vi "AlliGator Send Local Decay Plots.vi"(8 "error in (no error)":errorcluster, 10 "ROI Descriptor":T1 {"Contours"."Type" items=["No Selection", "Point", "Line", "Rectangle", "Oval", "Polygon", "Freehand Region", "Annulus", "Unused2", "Unused3", "Broken Line", "Freehand Line", "Rotated Rectangle"]}, 11 "AlliGator IV DVR in":refnum<data-value>) -> (0 "error out":errorcluster, 3 "AlliGator IV DVR out":refnum<data-value>)   [LabVIEW 2021, in "AlliGator Local Decay Window.lvlib"]
doc: "Gets the data (decay, fit, IRF, residuals and fit parameters) at the selected ROI and sends it to the Local Decay Window for update."
uses:
  AlliGator Local Decay Window.lvlib
  Internal Variables/AlliGator Internal Variables v2.ctl
  <vilib>/vision/Image Controls.llb/IMAQ Image.ctl
  Internal Variables/AlliGator Gate Image Set.ctl
  Files/AlliGator FLI Dataset Type.ctl
  Files/AlliGator Data Series Type.ctl
  Dual-Channel Datasets/AlliGator Dataset Channel.ctl
  Settings/AlliGator Gate Arithmetic.ctl
  Source Image/AlliGator Displayed Image.ctl
  Image/Named ROI Description.ctl
  Phasor Graph/AlliGator Decay Metadata v3.ctl
  Decay Analysis/Decay Preprocessing/AlliGator Decay Background Subtraction Info.ctl
  Decay Analysis/Decay Preprocessing/AlliGator Baseline Subtraction Method.ctl
  Graphs/XY Graph/XY Graph Plot Shift Parameters.ctl
  Graphs/XY Graph/XY Graph Plot Shift Method.ctl
  Decay Analysis/Decay Preprocessing/AlliGator Decay Extrapolation Parameters.ctl
  Phasor/Calibration Phasor (m, phi).ctl
  Phasor/Phasor Reference Series.ctl
  Phasor/Phasor Calibration Map v2.ctl
  Phasor/Phasor (g, s).ctl
  Phasor Graph/AlliGator Raw Phasor Plot Data v5.ctl
  Phasor/Phasor Standard Deviation Options.ctl
  Phasor Plot/AlliGator Phasor Multi-Harmonic Data.ctl
  Phasor/Phasor Harmonic Data.ctl
  Decay Fit Parameter Map/AlliGator Decay Fit Options & Parameters v4.ctl
  Fits/IRF(X)PSED/Decay Fit Options v4.ctl
  Fits/Decay Convolution/Decay Model.ctl
  Fits/Residual Type.ctl
  Fits/IRF(X)PSED/Fit Weights Type v2.ctl
  Fits/Non-linear Fitting Method v2.ctl
  Fits/Fit Calculation Method.ctl
  Fits/Non-linear Fitting Algorithm.ctl
  Decay Analysis/Decay Fit/AlliGator Decay Fit Parameter Constraints 2.ctl
  Fits/IRF(X)PSED/Decay Fit Parameters In List.ctl
  Fits/IRF(X)PSED/MLE Baseline Offset Type.ctl
  Decay Analysis/Decay Preprocessing/AlliGator Decay Preprocessing Parameters.ctl
  Fits/IRF(X)PSED/Decay Fit Parameters & Derived Quantities List v2.ctl
  Fits/IRF(X)PSED/Decay Fit Result Constraint.ctl
  Decay Fit Parameter Map/AlliGator Parameter Maps Data.ctl
  Globals, Variables, Constants/AlliGator Variables List.ctl
  AlliGator Local Decay Graph Window Event Refnum.ctl
  AlliGator Local Decay Fit Results.ctl
  Image Profile Window/AlliGator Image Profile Plot Data.ctl
  Graphs/XY Graph/XY Graph Plot Data.ctl
  Utilities/Read-Write.ctl
  Variant/Variant to Data/Variant to U16.vi
  Variant/Variant to Data/Variant to Boolean.vi
  Globals, Variables, Constants/AlliGator Globals, Variables & Constants.lvlib
  Graphs/XY Graph/XY Graph Add-Ons.lvlib
  Image Profile Window/AlliGator Image Profile Window.lvlib
  Decay Analysis/Decay Processing/AlliGator Decay Processing.lvlib
  Time/Time.lvlib
  Decay Fit Parameter Map/AlliGator Decay Fit Parameter Map.lvlib
  Decay Analysis/Decay Preprocessing/AlliGator Decay Preprocessing.lvlib
  GUI/AlliGator GUI.lvlib
  Utilities/Utilities.lvlib
  Variant/Variant to Data/Variant to Data.lvlib
  Image/Image.lvlib
  Fits/Fits.lvlib
  Phasor/Phasor.lvlib
  Internal Variables/AlliGator Internal Variables.lvlib
  Files/AlliGator Files.lvlib
  Phasor Graph/AlliGator Phasor Graph.lvlib
  Phasor Plot/AlliGator Phasor Plot.lvlib
  Source Image/AlliGator Source Image.lvlib
  Decay Analysis/Decay Fit/AlliGator Decay Fit.lvlib
  Settings/AlliGator Settings.lvlib
  Dual-Channel Datasets/AlliGator Dual-Channel Datasets.lvlib
panel:
  out "CPU (s)":dbl
  # "see the AlliGator License on the block diagram (Ctrl+E or Window:Show Block Diagram)"
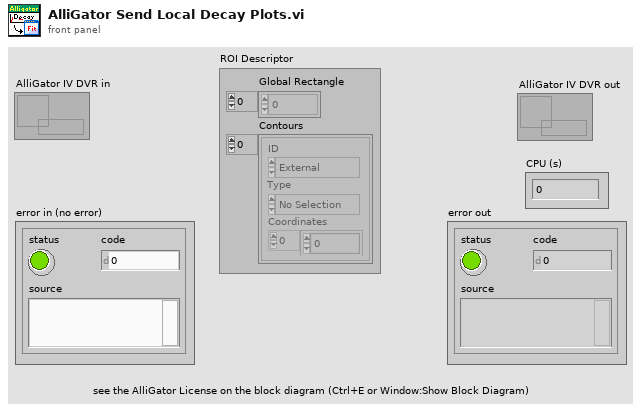
[diagram p1: front panel]
types:
  T1 = typedef "ROI Descriptor" = cluster{"Global Rectangle":i32[], "Contours":cluster{"ID":enum32{"External", "Internal"}, "Type":u32, "Coordinates":i32[]}[]}
  T2 = typedef "AlliGator Local Decay Window.lvlib/AlliGator Local Decay Graph Window Event Refnum.ctl" = refnum<user-event>
  T3 = typedef "AlliGator Globals, Variables & Constants.lvlib/AlliGator Variables List.ctl" = enum16{"---- GUI ----", "GUI:Initialization Status", "GUI:State Indicators Refnum", "GUI:Original AlliGator Menu Items", "GUI:Current Action Loop State", "GUI:Script in progress", "GUI:Playback", "GUI:Loop Playback", "GUI:Search ROI Used", "GUI:Search ROI", "Decay Graph Max Legend Size", "Intensity Graph Max Legend Size", "Decay Statistics Graph Max Legend Size", "Phasor Graph Max Legend Size", "Phasor Ratio Graph Max Legend Size", "Lifetime Graph Max Legend Size", "---- Files ----", "Files:Export Dataset Frames as Individual Files", "Files:Show Batch Export Help Balloons", "Files:Frames in Dataset", "Files:ptu File Frame Start Indices", "Files:Current Frame in Dataset", "Files:Current Frame Timestamp", "Files:Dataset Loaded", "Files:Dataset Metadata", "Files:Dataset Channel", "Files:Dataset Data Description", "Files:Background Dataset Metadata", "Files:Background Dataset Channel", "Files:Background Dataset Data Description", "Files:Background File Subtraction", "Files:Background File Path", "Files:Background File Pile-up Correction", "Files:Background File Pixel Well Capacity", "Files:Background File Scaling Factor", "Files:Current Dataset Load Settings", "Files:Dataset Path", "Files:ICCD-specific Information", "Files:Macrotime Gate Separation", "------ Python Plugins ------", "Python Plugins:Information", "Python Plugins:Python Session", "Python Plugins:Valid Python Session?", "---- Source Image ----", "Source Image:ROIs", "Source Image:Current ROI", "Source Image:ROI Event Refnum", "X_Source Image:Display Range", "X_Source Image:Palette Information", "X_Source Image:Type of Displayed Image", "X_Time Gate Slider", "Source Image:Palette List", "Source Image:Scale", "Source Image:ROI Overlay Color", "Source Image:Overlay to Erase", "Source Image:Is Displayed Image Accumulated", "Source Image:White Light Image Modified", "Source Image:Mask Image Modified", "---- Image Profile Window ----", "Image Profile:Window Event Refnum", "Image Profile:IntensityType", "Image Profile:Intensity Average Type", "Image Profile:Intensity-weighted SDV", "Image Profile:Box Profile Type", "Image Profile:Window Open", "Image Profile:Plotted Fit Parameter", "------ Phasor Graph -------", "Phasor Graph:Show Line", "---- Phasor Plot ---", "Phasor Plot:Parameters Changed", "Phasor Plot:FLI Dataset Modified since last Calculation", "Phasor Harmonics Data", "Selected Phasor Harmonics", "Phasor Harmonic Manager Event Refnum", "Phasor Plot:ROIs", "Phasor Plot:Current ROI", "Phasor Plot:ROI Event Refnum", "Phasor Plot:Image Reference Points", "Phasor Plot:Computed", "Phasor Plot:Palette Information", "Phasor Plot:Palette List", "Phasor Plot:Phasor Ratio Palette Information", "Phasor Plot:Phasor Ratio Palette List", "Phasor Plot:Image Scale", "Phasor Plot:Image Overlay to Erase", "Phasor Plot:Image Elements to Update", "Phasor Plot:Current Calculation Parameters", "Phasor Plot:Current Calibration Options", "Phasor Plot:Reset Cumulated Phasor Plot", "Phasor Plot:Reference 1", "Phasor Plot:Lifetime Reference 1", "Phasor Plot:Reference 1 Frequency", "Phasor Plot:Reference 2", "Phasor Plot:Lifetime Reference 2", "Phasor Plot:Reference 2 Frequency", "---- Decay Analysis ----", "Number of Selected Decays to Fit", "LS Fit Results", "LAR Fit Results", "BS Fit Results", "Last Decay Max - Min", "Best Fit Parameters", "Best Fit Parameter Names", "Actual Size X", "Actual Size Y", "Binning X", "Binning Y", "Actual # Gates", "Dataset Number", "Gates to...", "Gates Skipped", "Gates to keep", "Gate Step", "Gate Separation", "Reversed Gates", "Pile-up Correction", "Pixel Well Capacity", "Background Subtracted", "Background Subtraction Method", "Background Definition Range", "Background File (deprecated)", "Number of Dataset Accumulated", "Array of Accumulated Dataset Paths", "Do Averaged Datasets", "Destination File Path", "Process Plot Target", "Use 1/D as Phasor Frequency", "---- Decay Fit Parameter Map -----", "Decay Fit Parameter Map:Palette Information", "Decay Fit Parameter Map:Palette List", "Decay Fit Parameter Map:X Resolution", "Decay Fit Parameter Map:Y Resolution", "Decay Fit Parameter Map:Use Decay Fit Result Constraints", "Decay Fit Parameter Map:Decay Fit Result Constraints", "Decay Fit Parameter Map:Decay Fit Result Constraints Applied", "---- Parameter Map ----", "Parameter Map:Palette Information", "Parameter Map:Palette List", "------- Local Decay Window ---------", "Local Decay Graph Window:Event Refnum", "Local Decay Graph Window:Use normalized IRF for convolution", "----- Miscellaneous ----", "Misc:Skippable Dialog Windows Status"}
  T4 = typedef "IMAQ Image.ctl" = refnum<image>
  T5 = typedef "AlliGator Image Profile Window.lvlib/AlliGator Image Profile Plot Data.ctl" = cluster{"Plot Name":string, "Plot":T6}
  T6 = typedef "XY Graph Add-Ons.lvlib/XY Graph Plot Data.ctl" = cluster{"X Array":dbl[], "Y Array":dbl[]}
  T7 = typedef "AlliGator Internal Variables.lvlib/AlliGator Internal Variables v2.ctl" = cluster{"----------------------------- Images -----------------------------":u8, "Displayed Image":T4, "White Light Image":T4, "Mask Image":T4, "ROI Mask Image":T4, "Current Dataset Images 1":T8, "Background Dataset Images 1":T8, "Current Dataset Images 2":T8, "Background Dataset Images 2":T8, "Current Dataset Arithmetic Images":T8, "Accumulated Dataset Images 1":T8, "Accumulated Dataset Images 2":T8, "Accumulated Dataset Arithmetic Images":T8, "----------------------------- File Paths -----------------------------":u8, "Phasor Plot Image":T4, "Decay Fit Parameter Map Image":T4, "Parameter Map Image":T4, "Single Data Point Path":path, "White Light Image Path":path, "Mask Image Path":path, "Time-Series Folder":path, "[Time-Series Paths]":path[], "----------------------------- FLI Dataset -----------------------------":u8, "Current Dataset":i32, "Single Dataset Type":T9, "Current Folder":string, "AlliGator Data Series Type":T10, "# Datasets":i32, "Dual-Channel Dataset":bool, "Selected Channel Name":string, "Dataset Channel":T11, "Channel Arithmetic":T12, "Dual-Channel Background Dataset":bool, "Background Channel":T11, "Dual-Channel Accumulated Dataset":bool, "Start Time":dbl, "[Time-Series Timestamps]":dbl[], "[Intensity Corrections]":dbl[], "Time Series Script":bool, "Type of Displayed Image":T13, "Gate Image Slide":u16, "# Gates":i32, "ROIs":T14[], "----------------------------- Decays -----------------------------":u8, "ROI Decay":cluster{"t Array":dbl[], "I Array":dbl[]}, "Valid Decay":bool, "Decay  Metadata":T15, "Reference Decay Plot Name":string, "Reference Decay":cluster{"t Array":dbl[], "I Array":dbl[]}, "Decay Shift Plot":cluster{"Time Stamps":dbl[], "Decay Shifts":dbl[]}, "[Decays Max Values]":sgl[], "[Decays Min Values]":sgl[], "----------------------------- Calibration -----------------------------":u8, "Calibration Phasor":T21, "Calibration Phasor Series":T22, "Phasor Calibration Map":T23, "Calibration Map MD5 Digest":string, "----------------------------- Phasor Graph -----------------------------":u8, "Last Raw Phasor":T24, "Last Calibrated Phasor":T24, "Last Calibrated Phasor SDV":T24, "Phasor Graph:Phasor Plot":cluster{"g Array":dbl[], "s Array":dbl[]}, "Phasor Graph:Phasor SDV Plot":cluster{"g Array":dbl[], "s Array":dbl[]}, "[Phasor Graph:Raw Phasor Plots]":T25[], "Phasor Plot locked to Ref 1":i32, "[Phasor Plot(s) locked to Ref 1]":i32[], "[Phasor Plot(s) locked to Ref 2]":i32[], "[Pixel Phasors]":T24[], "----------------------------- Phasor Plot -----------------------------":u8, "[[Sum Image]]":dbl[][], "[[CSG Phasors]]":csg[][], "[[Valid Pixel?]]":bool[][], "[[Phasor Ratios]]":dbl[][], "[[Average Lifetimes]]":dbl[][], "Amplitude Weighted Average Lifetime":bool, "I/m/phi Dataset":cluster{"I/m/phi Dataset?":bool, "Base Frequency":dbl[unit], "Harmonic Orders":u8[]}, "Multi Phasor Plot Data":T27, "----------------------------- Decay Fit Parameter Map -----------------------------":u8, "Decay Fit Options & Parameters":T29, "Fit Options: Decay Preprocessing Parameters":T40, "Fit Options: Reference Decay":cluster{"t Array":dbl[], "I Array":dbl[]}, "Is Full Image Parameters Map":bool, "Is Single-Pixels Parameters Map":bool, "NLSF Parameters Map X Resolution":i32, "NLSF Parameters Map Y Resolution":i32, "[Single Decay Fit Parameters]":dbl[], "Fit Model":T31, "[[Multiple Decays Fit Parameters]]":dbl[][], "[[Multiple Decays Fit Parameter SDVs]]":dbl[][], "[[IRFs]]":dbl[][], "[ROI Descriptors]":T1[], "IRF Array Time Axis":dbl[], "Decay Array Time Axis":dbl[], "[Decay Fit Parameter Names]":T41[], "[Decay Sum]":dbl[], "Array of Decay Fit Result Constraints":T42[], "Selected ROIs Array":bool[], "----------------------------- Parameter Maps -----------------------------":u8, "[Map Set Names]":string[], "[Parameter Maps]":T43[], "[[User-defined Quantities]]":dbl[][], "User-defined Quantity":string}
  T8 = typedef "AlliGator Internal Variables.lvlib/AlliGator Gate Image Set.ctl" = cluster{"SGL Gate Images":T4[], "SGL Sum Image":T4, "SGL Max Image":T4, "SGL Min Image":T4}
  T9 = typedef "AlliGator Files.lvlib/AlliGator FLI Dataset Type.ctl" = enum16{"HDF5 FLI Dataset", "Gate Image Folder", ".sdt FLI Dataset (Becker & Hickl)", ".ptu FLI Dataset (PicoQuant)", "SS1 FLI Dataset", "SS2 FLI Dataset", "I/m/phi Dataset", ".bin FLI Dataset (PicoQuant Binned)", ".bin FLI Dataset (Piccolo Binned)", ".mat FLI Dataset"}
  T10 = typedef "AlliGator Files.lvlib/AlliGator Data Series Type.ctl" = enum16{"Not a Supported Series", "Gate Images Folder Series", "SwissSPAD 2 Dataset Series", "B&H FLI Dataset Series", "PicoQuant PTU FLI Dataset Series", "PicoQuant BIN FLI Dataset Series", "Piccolo hist BIN FLI Dataset Series", "HDF5 FLI Dataset Series"}
  T11 = typedef "AlliGator Dual-Channel Datasets.lvlib/AlliGator Dataset Channel.ctl" = enum16{"G2", "INT"}
  T12 = typedef "AlliGator Settings.lvlib/AlliGator Gate Arithmetic.ctl" = enum16{"None", "INT-G2", "G2/INT*<INT>", "(1 - G2/INT)*<INT>"}
  T13 = typedef "AlliGator Source Image.lvlib/AlliGator Displayed Image.ctl" = enum16{"Single Gate", "Sum of All Gates", "Max of All Gates", "Min of All Gates", "-", "White Ligth Image", "Mask Image"}
  T14 = typedef "Image.lvlib/Named ROI Description.ctl" = cluster{"ROI Descriptor":T1, "ROI Name":string, "Overlay Color":u32}
  T15 = typedef "AlliGator Phasor Graph.lvlib/AlliGator Decay Metadata v3.ctl" = cluster{"ROI Descriptor":T1, "ROI Center":cluster{"X":i32, "Y":i32}, "Decay Background Subtraction Info":T16, "Decay Reverted":bool, "Decay Smoothened":bool, "Decay Straightened":bool, "Fitted Tau (Decay Straightening)":dbl, "Decay Shift Parameters":T18, "Decay Shifted":bool, "Decay Extrapolated":bool, "Decay Extrapolation Parameters":T20, "Decay Normalized":bool, "Fold Decay":bool, "# Folds":u32}
  T16 = typedef "AlliGator Decay Preprocessing.lvlib/AlliGator Decay Background Subtraction Info.ctl" = cluster{"Laser Period":dbl[unit], "Gate Duration":dbl[unit], "Baseline Subtraction Method":T17, "Background Definition Range":cluster{"Min Gate":dbl[unit], "Max Gate":dbl[unit]}, "Total Intensity w/o Bkgd Subtraction":dbl, "Bkgd-subtracted Intensity (exp)":dbl, "# Data Points":i32, "Background/Gate":dbl, "Fitted Lifetime":dbl[unit], "Bkgd-subtracted Intensity (theo)":dbl}
  T17 = typedef "AlliGator Decay Preprocessing.lvlib/AlliGator Baseline Subtraction Method.ctl" = enum16{"Mean", "Min", "Square Gated Single-Exponential", "File", "Constant"}
  T18 = typedef "XY Graph Add-Ons.lvlib/XY Graph Plot Shift Parameters.ctl" = cluster{"Type":T19, "Shift":dbl[unit], "Threshold":dbl, "Rotate":bool}
  T19 = typedef "XY Graph Add-Ons.lvlib/XY Graph Plot Shift Method.ctl" = enum16{"Default", "CFD", "Threshold", "Cross-Correlation"}
  T20 = typedef "AlliGator Decay Preprocessing.lvlib/AlliGator Decay Extrapolation Parameters.ctl" = cluster{"Additional Points":u32, "Head Fraction":dbl, "Fitted Tau":dbl, "Use Periodicity":bool, "Use Cursors":bool, "Tail Fraction":dbl}
  T21 = typedef "Phasor.lvlib/Calibration Phasor (m, phi).ctl" = cluster{"m":dbl, "phi":dbl, "Phasor Frequency":dbl[unit], "Reference Lifetime":dbl[unit]}
  T22 = typedef "Phasor.lvlib/Phasor Reference Series.ctl" = cluster{"m Array":dbl[], "phi Array":dbl[], "Phasor Frequency":dbl[unit], "Calibration Lifetime":dbl[unit]}
  T23 = typedef "Phasor.lvlib/Phasor Calibration Map v2.ctl" = cluster{"Phasor Frequency":dbl[unit], "Calibration Lifetime":dbl[unit], "ROI Centers":cluster{"X":i32, "Y":i32}[], "ROI Descriptors":T1[], "Map Resolution X":i32, "Map Resolution Y":i32, "z Array":cdb[]}
  T24 = typedef "Phasor.lvlib/Phasor (g, s).ctl" = cluster{"g":dbl, "s":dbl}
  T25 = typedef "AlliGator Phasor Graph.lvlib/AlliGator Raw Phasor Plot Data v5.ctl" = cluster{"Phasor Plot Name":string, "Raw Phasor Plot":T24[], "Phasor Frequency":dbl[unit], "[Decay Metadata]":T15[], "Raw Phasor Plot SDV":T24[], "Phasor SDV Options":T26, "[Calibration Phasor]":T21[], "Intensity Array":dbl[]}
  T26 = typedef "Phasor.lvlib/Phasor Standard Deviation Options.ctl" = cluster{"Compute Estimated SDV":bool, "# Replicas":u32, "Use Estimated Average Phasor":bool}
  T27 = typedef "AlliGator Phasor Plot.lvlib/AlliGator Phasor Multi-Harmonic Data.ctl" = cluster{"Base Frequency":dbl[unit], "# Harmonics":u8, "Harmonic Orders":u8[], "Phasor Plot Settings Checksum":u64, "Phasor Harmonic Data Array":T28[]}
  T28 = typedef "Phasor.lvlib/Phasor Harmonic Data.ctl" = cluster{"Phasor Harmonic Name":string, "Phasor Plot Settings Checksum":u64, "Phasor Frequency":dbl[unit], "Base Frequency":dbl[unit], "Harmonic Order":u8, "Phasor Plot Parameters":string, "Phasor Array [[CSG]]":csg[][], "Dataset File Path":path}
  T29 = typedef "AlliGator Decay Fit Parameter Map.lvlib/AlliGator Decay Fit Options & Parameters v4.ctl" = cluster{"SYNC Period":dbl[unit], "Fit Options":T30, "Fit Parameter Constraints":T37[], "MLE Baseline Offset":dbl, "MLE Baseline Offset Type":T39}
  T30 = typedef "Fits.lvlib/Decay Fit Options v4.ctl" = cluster{"Show Fit Residuals":bool, "Fit Model":T31, "Residual Type":T32, "Max Decay Percentile":dbl, "Min Decay Percentile":dbl, "Show Full Decay":bool, "Weights":T33, "Fitting Method":T34, "Compute Parameter Uncertainties":bool, "Periodic Boundaries":bool, "Model Calculation":T35, "Period":dbl[unit], "Termination Criteria":cluster{"Max Iterations":i32, "Max Function Calls":i32, "Max Time":dbl[unit], "Function Tolerance":dbl, "Parameter Tolerance":dbl, "Gradient Tolerance":dbl, "Min Lambda":dbl, "Max Lambda":dbl, "Initial Tick Count":u32}, "Offset Resolution":dbl[unit], "Use Local IRF":bool, "Fitting Algorithm":T36, "Show Confidence Interval ":bool, "Confidence Level":dbl}
  T31 = typedef "Fits.lvlib/Decay Model.ctl" = enum16{"1-Exponential", "2-Exponentials"}
  T32 = typedef "Fits.lvlib/Residual Type.ctl" = enum16{"Standard", "Normalized", "Reduced"}
  T33 = typedef "Fits.lvlib/Fit Weights Type v2.ctl" = enum16{"Unweighted", "1/Variance (Neyman)", "1/Variance (Pearson)", "Best of All"}
  T34 = typedef "Fits.lvlib/Non-linear Fitting Method v2.ctl" = enum16{"Least Square", "Least Absolute Residual", "Bisquare", "MLE", "-", "Best of All"}
  T35 = typedef "Fits.lvlib/Fit Calculation Method.ctl" = enum16{"Simulation", "Convolution", "Integration"}
  T36 = typedef "Fits.lvlib/Non-linear Fitting Algorithm.ctl" = enum16{"Levenberg-Marquardt", "Trust-Region Dogleg"}
  T37 = typedef "AlliGator Decay Fit.lvlib/AlliGator Decay Fit Parameter Constraints 2.ctl" = cluster{"Fit Parameter":T38, "Min Value":dbl, "Max Value":dbl, "Global":bool, "Used":bool}
  T38 = typedef "Fits.lvlib/Decay Fit Parameters In List.ctl" = enum16{"Offset", "Baseline", "A_1", "tau_1", "A_2", "tau_2"}
  T39 = typedef "Fits.lvlib/MLE Baseline Offset Type.ctl" = enum32{"Absolute", "Percentage"}
  T40 = typedef "AlliGator Decay Preprocessing.lvlib/AlliGator Decay Preprocessing Parameters.ctl" = cluster{"Background Subtraction":bool, "Straighten Decay":bool, "Reverse Gates":bool, "1-Normalized Decay":bool, "Smoothen Decay":bool, "Smoothing Parameter":dbl, "Shift Decay":bool, "Decay Shift Parameters":T18, "Extrapolate Decay":bool, "Additional Points":u32, "Head Fraction":dbl, "Pixel-Normalize Decay":bool, "Use Periodicity":bool, "Use Cursors":bool, "Tail Fraction":dbl, "Use Decay Pre-Processing":bool, "Fold Decay":bool, "# Folds":u32, "[0-1]-Normalized Decay":bool}
  T41 = typedef "Fits.lvlib/Decay Fit Parameters & Derived Quantities List v2.ctl" = enum16{"Offset", "Baseline", "A_1", "tau_1", "A_2", "tau_2", "<tau>_a", "f1_a", "f2_a", "<tau>_i", "f1_i", "f2_i", "-", "R^2", "Chi^2"}
  T42 = typedef "Fits.lvlib/Decay Fit Result Constraint.ctl" = cluster{"Fit Parameter":enum16{"Offset", "Baseline", "A_1", "tau_1", "A_2", "tau_2", "<tau>_a", "f1_a", "f2_a", "<tau>_i", "f1_i", "f2_i", "-", "R^2", "Chi^2", "Max Relative Residual", "<Residual ACF>", "Residual ACF SDV", "tau_2/tau_1"}, "Min Value":dbl, "Max Value":dbl, "Use Constraint":bool}
  T43 = typedef "AlliGator Decay Fit Parameter Map.lvlib/AlliGator Parameter Maps Data.ctl" = cluster{"Map Set Name":string, "[Parameter Names]":string[], "[[Parameters]]":dbl[][], "[[Parameter SDVs]]":dbl[][], "Decay Array Time Axis":dbl[], "[[IRFs]]":dbl[][], "IRF Array Time Axis":dbl[], "X Resolution":i32, "Y Resolution":i32, "Intensity Array":dbl[]}
  T44 = cluster{"IRF Array Time Axis":dbl[], "[[IRFs]]":dbl[]}
  T45 = cluster{"t Axis":dbl[], "ROI Intensity Array":dbl[]}
  T46 = typedef "Utilities.lvlib/Read-Write.ctl" = enum16{"Read", "Write"}
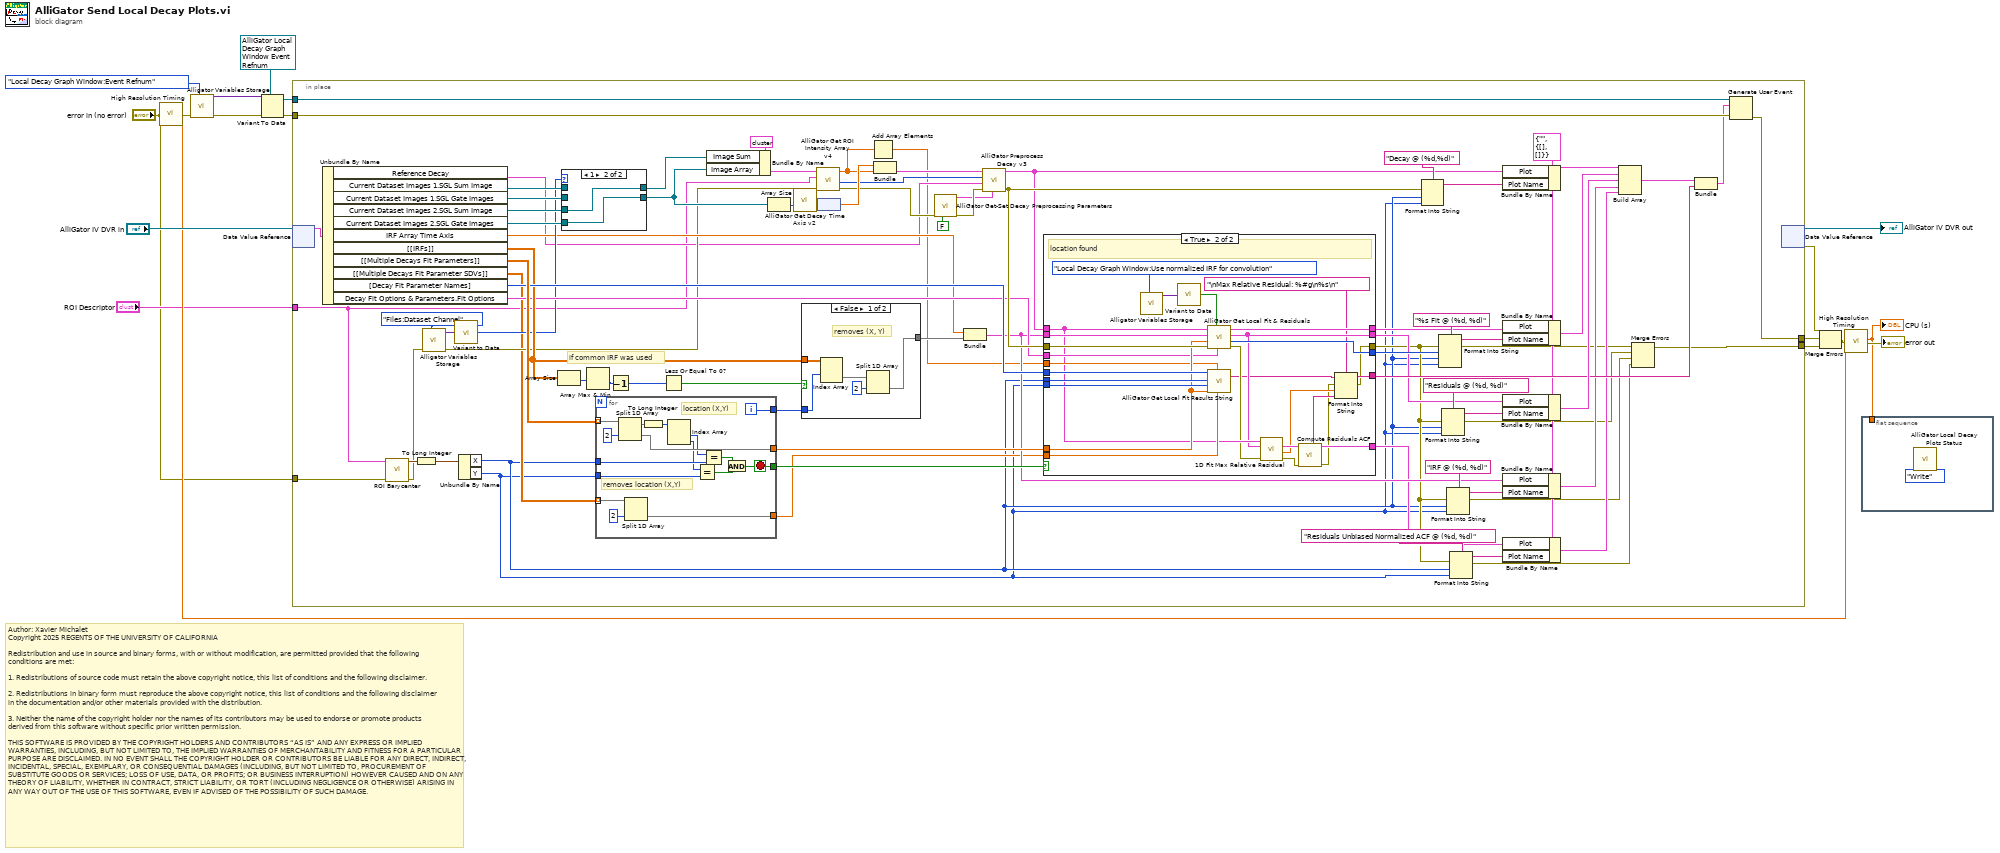
[diagram p0: block diagram]
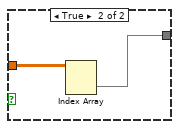
[diagram p3: hidden frame]
diagram:
  # "Author: Xavier Michalet\nCopyright 2025 REGENTS OF THE UNIVERSITY OF CALIFORNIA\n\nRedistribution and use in source and binary forms, with or without modification, are permitted provided that the following conditions are met:\n\n1. Redistributions of source code must retain the above copyright notice, this list of conditions and the following disclaimer.\n\n2. Redistributions in binary form must reproduce the above copyright notice, this list of conditions and the following disclaimer in the documentation and/or other materials provided with the distribution.\n\n3. Neither the name of the copyright holder nor the names of its contributors may be used to endorse or promote products derived from this software without specific prior written permission.\n\nTHIS SOFTWARE IS PROVIDED BY THE COPYRIGHT HOLDERS AND CONTRIBUTORS “AS IS” AND ANY EXPRESS OR IMPLIED WARRANTIES, INCLUDING, BUT NOT LIMITED TO, THE IMPLIED WARRANTIES OF MERCHANTABILITY AND FITNESS FOR A PARTICULAR PURPOSE ARE DISCLAIMED. IN NO EVENT SHALL THE COPYRIGHT HOLDER OR CONTRIBUTORS BE LIABLE FOR ANY DIRECT, INDIRECT, INCIDENTAL, SPECIAL, EXEMPLARY, OR CONSEQUENTIAL DAMAGES (INCLUDING, BUT NOT LIMITED TO, PROCUREMENT OF SUBSTITUTE GOODS OR SERVICES; LOSS OF USE, DATA, OR PROFITS; OR BUSINESS INTERRUPTION) HOWEVER CAUSED AND ON ANY THEORY OF LIABILITY, WHETHER IN CONTRACT, STRICT LIABILITY, OR TORT (INCLUDING NEGLIGENCE OR OTHERWISE) ARISING IN ANY WAY OUT OF THE USE OF THIS SOFTWARE, EVEN IF ADVISED OF THE POSSIBILITY OF SUCH DAMAGE."
  n1 = call "High Resolution Timing.vi"("Error In"="error in (no error)") -> ("elapsed (relative) seconds"=w6:dbl, "Error Out"=w9:errorcluster)  [unwired: 16 in, 1 out]
  n2 = call "Alligator Variables Storage.vi"("AlliGator Variable"=AlliGator_Variables_List."Local Decay Graph Window:Event Refnum" ("Alligator Variable"), "Error In"=w9) -> ("Error Out"=w15:errorcluster, "Data out"=w13:variant)  [unwired: 7 in, 1 out]
  n3 = Variant To Data(error in=w15, type=T2 refnum ("Local Decay Graph Window Event Refnum"), Variant=w13) -> (data=w11:T2, error out=w14:errorcluster)
  n4 = in-place {
    in-place-border: w14 -> [w97]
    in-place-border: w11 -> [w99]
    in-place-border: [w98] -> w10
    in-place-border: "ROI Descriptor" -> [w22]
    in-place-border: [w29] -> w5
    in-place-border: "error in (no error)" -> [w23]
    w34 = T5 {"Plot Name"="", "Plot"={"X Array"=[], "Y Array"=[]}} ("Plot Data")
    # "if common IRF was used"
    n5 = in-place-dvr #1("AlliGator IV DVR in") -> (w100:T7)  [unwired: 1 out]
    n6 = Unbundle By Name(w100) -> ("Reference Decay"=w41:cluster{"t Array":dbl[], "I Array":dbl[]}, "Current Dataset Images 1.SGL Sum Image"=w60:T4, "Current Dataset Images 1.SGL Gate Images"=w63:T4[], "Current Dataset Images 2.SGL Sum Image"=w59:T4, "Current Dataset Images 2.SGL Gate Images"=w62:T4[], "IRF Array Time Axis"=w47:dbl[], "[[IRFs]]"=w53:dbl[][], "[[Multiple Decays Fit Parameters]]"=w81:dbl[][], "[[Multiple Decays Fit Parameter SDVs]]"=w38:dbl[][], "[Decay Fit Parameter Names]"=w78:T41[], "Decay Fit Options & Parameters.Fit Options"=w51:T30)
    n7 = call "ROI Barycenter.vi"("Error In"=w23, "ROI Descriptor in"=w22) -> ("Error Out"=w21:errorcluster, "ROI Center"=w24:cluster{"X":dbl, "Y":dbl})  [unwired: 7 in, 1 out]
    n8 = To Long Integer(number=w24) -> (32bit integer=w25:cluster{"X":i32, "Y":i32})
    n9 = call "Alligator Variables Storage.vi"("AlliGator Variable"=AlliGator_Variables_List."Files:Dataset Channel" ("Alligator Variable"), "Error In"=w21) -> ("Error Out"=w42:errorcluster, "Data out"=w49:variant)  [unwired: 7 in, 1 out]
    n10 = call-poly "Variant to Data.vi"("Variant"=w49) -> ("U16 Value"=w48:u16)  [unwired: 8 in]
    n11 = Unbundle By Name(w25) -> ("X"=w20:i32, "Y"=w19:i32)
    n12 = Array Size(array=w53) -> (size(s)=w57:i32[])
    n13 = case shown="1" w48 {
      tunnel: [w102 w104] -> w58
      tunnel: w59 -> [_ w104]
      tunnel: w62 -> [_ w103]
      tunnel: [w101 w103] -> w61
      tunnel: w60 -> [w102 _]
      tunnel: w63 -> [w101 _]
      frame 0, Default {
      }
      frame 1 {
      }
    }
    n14 = Array Max & Min(array=w57) -> (min value=w56:i32)  [unwired: 3 out]
    n15 = for {
      tunnel: w81 -> [w155] mode=indexing
      tunnel: w20 -> [w154]
      tunnel: w19 -> [w153]
      tunnel: [w152] -> w87
      tunnel: [w151] -> w82
      tunnel: [w145] -> w52
      tunnel: w38 -> [w142] mode=indexing
      tunnel: [w140] -> w37
      i -> [w145]
      stop <- w152 stop-if-true
      # "location (X,Y)"
      # "removes location (X,Y)"
      n16 = Split 1D Array(array=w155, index=2) -> (first subarray=w144:dbl[], second subarray=w151:dbl[])
      n17 = Split 1D Array(array=w142, index=2) -> (second subarray=w140:dbl[])  [unwired: 1 out]
      n18 = To Long Integer(number=w144) -> (32bit integer=w143:i32[])
      n19 = Index Array(array=w143) -> (element #1=w149:i32, element #2=w148:i32)  [unwired: 2 in]
      n20 = Equal?(x=w148, y=w153) -> (x = y?=w146:bool)
      n21 = Equal?(x=w149, y=w154) -> (x = y?=w147:bool)
      n22 = And(x=w147, y=w146) -> (x .and. y?=w152:bool)
    }
    n23 = Decrement(x=w56) -> (x-1=w55:i32)
    n24 = Less Or Equal To 0?(x=w55) -> (x <= 0?=w54:bool)
    n25 = Bundle By Name(cluster=cluster{"Image Sum":T4, "Image Array":T4[]} {"Image Sum"=refnum, "Image Array"=[]} ("Images"), "Image Sum"=w58, "Image Array"=w61) -> (w85:cluster{"Image Sum":T4, "Image Array":T4[]})
    n26 = Array Size(array=w61) -> (size(s)=w84:i32)
    n27 = call "AlliGator Get Decay Time Axis v2.vi"("Number of Gates"=w84) -> ("t Array"=w83:dbl[unit][])  [unwired: 14 in]
    n28 = case shown="False" w54 {
      tunnel: w53 -> [w109 w111]
      tunnel: [w106 w110] -> w46
      tunnel: w52 -> [w108 _]
      frame False {
        # "removes (X, Y)"
        n29 = Index Array(array=w109, index (row)=w108) -> (element=w107:dbl[])  [unwired: 1 in]
        n30 = Split 1D Array(array=w107, index=2) -> (second subarray=w106:dbl[])  [unwired: 1 out]
      }
      frame True {
        n31 = Index Array(array=w111) -> (element=w110:dbl[])  [unwired: 2 in]
      }
    }
    n32 = call "AlliGator Get ROI Intensity Array v4.vi"("error in (no error)"=w42, "ROI Descriptor"=w22, "Images"=w85) -> ("Error Out"=w71:errorcluster, "# Valid Pixels"=w69:i32, "ROI Intensity Array"=w40:dbl[])  [unwired: 3 in, 3 out]
    n33 = node(w83) -> (w80:dbl[])
    n34 = Add Array Elements(numeric array=w40) -> (sum=w39:dbl)
    n35 = Bundle(w80, "ROI Intensity Array"=w40) -> (w68:cluster{dbl[], "ROI Intensity Array":dbl[]})  [unwired: 1 in]
    n36 = call "AlliGator Get-Set Decay Preprocessing Parameters.vi"("Get (F)/Set"=FALSE, "Error In"=w71) -> ("Error Out"=w70:errorcluster, "Decay Preprocessing Parameters out"=w66:T40)  [unwired: 8 in]
    n37 = Bundle("IRF Array Time Axis"=w47, "[[IRFs]]"=w46) -> (w43:T44)  [unwired: 1 in]
    n38 = call "AlliGator Preprocess Decay v3.vi"("Decay Preprocessing Parameters"=w66, "Error In"=w70, "Time-Gated Reference Decay"=w41, "# Pixels"=w69, "Decay (in)"=w68) -> ("Error Out"=w67:errorcluster, "Decay (out)"=w64:T45)  [unwired: 3 in, 2 out]
    n39 = case shown="True" w87 {
      tunnel: w82 -> [_ w134]
      tunnel: w67 -> [w112 w139]
      tunnel: [w112 w114] -> w31
      tunnel: w64 -> [_ w124]
      tunnel: [_ w138] -> w79
      tunnel: w78 -> [_ w137]
      tunnel: w20 -> [_ w136]
      tunnel: w19 -> [_ w135]
      tunnel: [_ w116] -> w76
      tunnel: w51 -> [_ w133]
      tunnel: w43 -> [_ w132]
      tunnel: [_ w131] -> w45
      tunnel: [_ w121] -> w44
      tunnel: w39 -> [_ w127]
      tunnel: w37 -> [_ w126]
      tunnel: [_ w125] -> w32
      frame False {
        # "Not a valid location"
      }
      frame True {
        # "location found"
        n40 = call "Alligator Variables Storage.vi"("AlliGator Variable"=AlliGator_Variables_List."Local Decay Graph Window:Use normalized IRF for convolution") -> ("Data out"=w130:variant)  [unwired: 8 in, 2 out]
        n41 = call-poly "Variant to Data.vi"("Variant"=w130) -> ("Value"=w128:bool)  [unwired: 8 in]
        n42 = call "AlliGator Get Local Fit & Residuals.vi"("Fit Options"=w133, "Use Normalized IRF (T)"=w128, "Error In"=w139, "All Fit Parameters (w tau)"=w134, "IRF"=w132, "Decay Plot"=w124) -> ("Error Out"=w123:errorcluster, "Fit Model"=w138:T31, "Residual Plot"=w121:cluster{"X Array":dbl[], "Y Array":dbl[]}, "Fit Plot"=w131:cluster{"X Array":dbl[], "Y Array":dbl[]})  [unwired: 2 in]
        n43 = call "AlliGator Get Local Fit Results String.vi"("Parameters SDV"=w126, "Decay Sum"=w127, "Parameters"=w134, "Y"=w135, "X"=w136, "[Decay Fit Parameter Name]"=w137) -> ("Fit Results String"=w119:string)  [unwired: 5 in]
        n44 = call "1D Fit Max Relative Residual.vi"("error in (no error)"=w123, "Residual Plot"=w121, "Plot"=w124) -> ("error out"=w122:errorcluster, "Max Relative Residual"=w117:dbl, "Residual Plot (dup)"=w120:cluster{"X Array":dbl[], "Y Array":dbl[]})  [unwired: 6 in]
        n45 = call "Compute Residuals ACF.vi"("Error In"=w122, "Residual Plot in"=w120) -> ("Error Out"=w115:errorcluster, "Residual ACF out"=w125:cluster{"X Array":dbl[], "Y Array":dbl[]}, "ACF Statistics"=w118:string)  [unwired: 5 in, 2 out]
        n46 = Format Into String(format string="\nMax Relative Residual: %#g\n%s\n", initial string=w119, error in=w115, w117, w118) -> (resulting string=w116:string, error out=w114:errorcluster)
      }
    }
    n47 = Format Into String(format string="Decay @ (%d,%d)" ("Plot Name"), error in=w67, w20, w19) -> (resulting string=w93:string)  [unwired: 1 in, 1 out]
    n48 = Format Into String(format string="%s Fit @ (%d, %d)" ("Plot Name"), error in=w31, w79, w20, w19) -> (resulting string=w90:string, error out=w30:errorcluster)  [unwired: 1 in]
    n49 = Format Into String(format string="Residuals @ (%d, %d)" ("Plot Name"), error in=w31, w20, w19) -> (resulting string=w88:string, error out=w28:errorcluster)  [unwired: 1 in]
    n50 = Format Into String(format string="IRF @ (%d, %d)" ("Plot Name"), error in=w31, w20, w19) -> (resulting string=w73:string, error out=w27:errorcluster)  [unwired: 1 in]
    n51 = Format Into String(format string="Residuals Unbiased Normalized ACF @ (%d, %d)" ("Plot Name"), error in=w31, w20, w19) -> (resulting string=w35:string, error out=w26:errorcluster)  [unwired: 1 in]
    n52 = Bundle By Name(cluster=w34, "Plot"=w64, "Plot Name"=w93) -> (w96:T5)
    n53 = Bundle By Name(cluster=w34, "Plot"=w45, "Plot Name"=w90) -> (w95:T5)
    n54 = Bundle By Name(cluster=w34, "Plot"=w44, "Plot Name"=w88) -> (w94:T5)
    n55 = Bundle By Name(cluster=w34, "Plot"=w43, "Plot Name"=w73) -> (w72:T5)
    n56 = Bundle By Name(cluster=w34, "Plot"=w32, "Plot Name"=w35) -> (w33:T5)
    n57 = Build Array(w96, w95, w94, w72, w33) -> (w77:T5[])
    n58 = Merge Errors(w30, w28, w27, w26) -> (w29:errorcluster)
    n59 = Bundle(w77, w76) -> (w75:cluster{T5[], string})  [unwired: 1 in]
    n60 = Generate User Event(user event=w99, event data cluster=w75, error in=w97) -> (error out=w98:errorcluster)  [unwired: 1 in, 1 out]
    n61 = in-place-dvr #1() -> (→"AlliGator IV DVR out":refnum<data-value>, w4:errorcluster)  [unwired: 1 in]
  }
  n62 = Merge Errors(w4, w10, w5) -> (w8:errorcluster)
  n63 = call "High Resolution Timing.vi"("relative seconds (NaN)"=w6, "Error In"=w8) -> ("elapsed (relative) seconds"=w1:dbl, "Error Out"=→"error out":errorcluster)  [unwired: 15 in, 1 out]
  "CPU (s)" <- w1
  n64 = flat-sequence {
    tunnel: w1 -> [_]
    frame #0 {
      n65 = call "AlliGator Local Decay Plots Status.vi"("Read/Write"=Read-Write."Write") -> ()  [unwired: 8 in, 1 out]
    }
  }
